vi "Read configuration.vi"(8 "error in":errorcluster, 11 "OPC UA editor node in":refnum<class "OPC UA Server editor node.lvclass">) -> (0 "error out":errorcluster, 2 "configuration":refnum<class "NISE_CEF_serializable configuration.lvclass">, 3 "OPC UA editor node out":refnum<class "OPC UA Server editor node.lvclass">)   [LabVIEW 2013, in "OPC UA Server editor node.lvclass"]
uses:
  OPC UA Server editor node.lvclass
  <vilib>/NI/Configuration Framework/serializable configuration/NISE_CEF_serializable configuration.lvclass
  OPC UA Server editor node.lvclass/OPC UA Server editor node.ctl
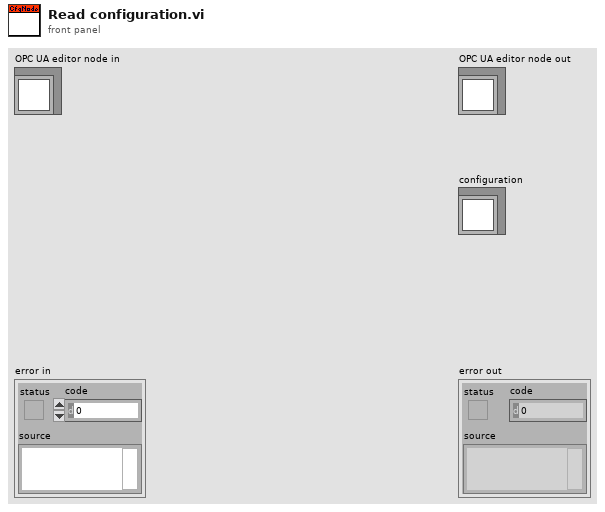
[diagram p1: front panel]
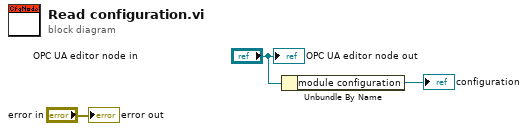
[diagram p0: block diagram]
diagram:
  n1 = Unbundle By Name("OPC UA editor node in") -> ("module configuration"=→"configuration":refnum<class "OPC UA Server configuration.lvclass">)
  "error out" <- "error in"
  "OPC UA editor node out" <- "OPC UA editor node in"
